vi "Calculation_test.vi"() -> (0 "New Values In":string[][](array[string])=[["Test data5"]], 1 "New Chs In":string[](array[string])=["30-10-03:New:Channel new5"])   [LabVIEW 2010]
uses:
  Results_plotter_Global.vi
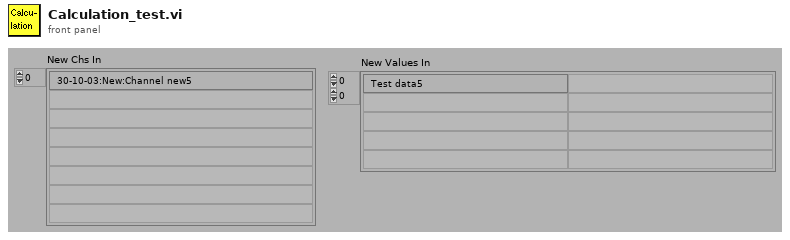
[diagram p1: front panel]
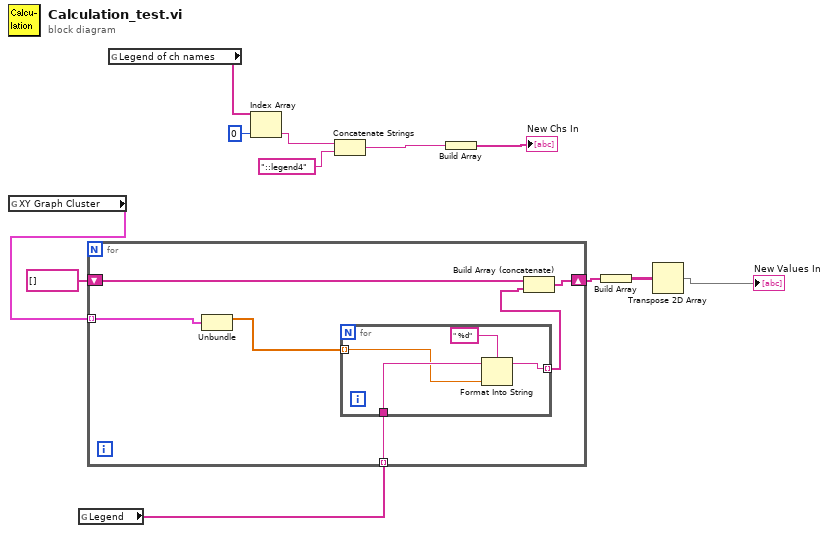
[diagram p0: block diagram]
diagram:
  n1 = global read "Results_plotter_Global.vi" "XY Graph Cluster"() -> (w9:cluster{dbl[], dbl[]}[])
  n2 = global read "Results_plotter_Global.vi" "Legend"() -> (w1:string[])
  n3 = for {
    tunnel: w9 -> [w18] mode=indexing
    shift-right: [w16] -> w7
    shift-left: string[] [] -> [w15]
    tunnel: w1 -> [w14] mode=indexing
    n4 = Unbundle(w18) -> (w13:dbl[])  [unwired: 1 out]
    n5 = for {
      tunnel: [w20] -> w17 mode=indexing
      tunnel: w14 -> [w22]
      tunnel: w13 -> [w21] mode=indexing
      n6 = Format Into String(format string=" %d", initial string=w22, w21) -> (resulting string=w20:string)  [unwired: 1 in, 1 out]
    }
    n7 = Build Array (concatenate)(w15, w17) -> (w16:string[])
  }
  n8 = global read "Results_plotter_Global.vi" "Legend of ch names"() -> (w4:string[])
  n9 = Index Array(array=w4, index=0) -> (element=w2:string)
  n10 = Concatenate Strings(w2, "::legend4" ("string")) -> (w11:string)
  n11 = Build Array(w11) -> (→"New Chs In":string[])
  n12 = Build Array(w7) -> (w6:string[][])
  n13 = Transpose 2D Array(2D array=w6) -> (transposed array=→"New Values In":string[][])
